vi "readConfigData.vi"(6 "Section":string, 7 "error in":errorcluster, 10 "refnum":T1) -> (0 "error out":errorcluster, 2 "Array":string[][](array[string]), 3 "refnum out":T1)   [LabVIEW 2014]
uses:
  <vilib>/Utility/config.llb/Config Data RefNum.ctl
  <vilib>/Utility/config.llb/Read Key (String).vi
  <vilib>/Utility/config.llb/NI_LVConfig.lvlib
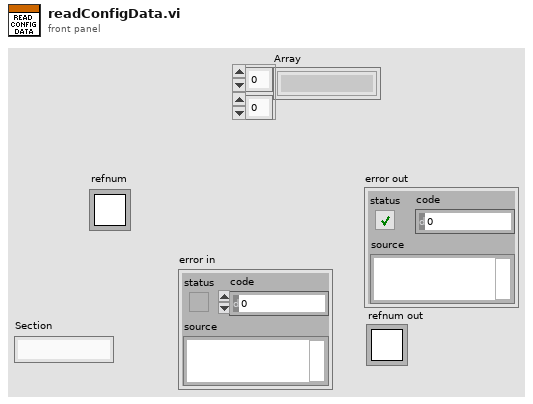
[diagram p1: front panel]
types:
  T1 = typedef "NI_LVConfig.lvlib/Config Data RefNum.ctl" = refnum<k1>
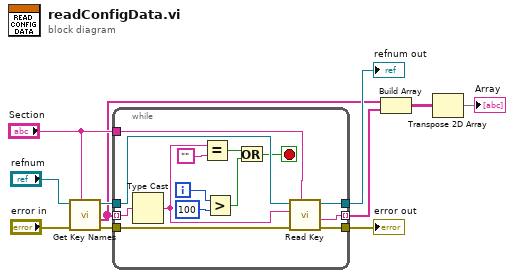
[diagram p0: block diagram]
diagram:
  n1 = call <vilib>:"Get Key Names.vi"("section"="Section", "error in (no error)"="error in", "refnum"="refnum") -> ("error out"=w7:errorcluster, "key names"=w4:string[], "refnum out"=w8:T1)  [unwired: 5 in, 1 out]
  n2 = while {
    tunnel: w4 -> [w25] mode=indexing
    tunnel: w8 -> [w24]
    tunnel: [w23] -> w3 mode=indexing
    tunnel: [w22] -> w10
    tunnel: [w21] -> w11
    tunnel: "Section" -> [w20]
    tunnel: w7 -> [w12]
    i -> [w17]
    stop <- w15 stop-if-true
    n3 = Type Cast(x=w25) -> (*(type *) &x=w18:string)  [unwired: 1 in]
    n4 = Equal?(x=w18, y="") -> (x = y?=w14:bool)
    n5 = Greater?(x=w17, y=100) -> (0:w13:bool)
    n6 = Or(x=w14, y=w13) -> (x .or. y?=w15:bool)
    n7 = call-poly <vilib>:"Read Key.vi"("section"=w20, "error in (no error)"=w12, "key"=w18, "refnum"=w24) -> ("error out"=w21:errorcluster, "value"=w23:string, "refnum out"=w22:T1)  [unwired: 4 in, 1 out]
  }
  "error out" <- w11
  "refnum out" <- w10
  n8 = Build Array(w4, w3) -> (w2:string[][])
  n9 = Transpose 2D Array(2D array=w2) -> (transposed array=→"Array":string[][])
